vi "Call_enqueue_small.vi"(7 "Waveform":T6(array[cluster])=[{"first point time"=-0.004999939551282051, "xIncrement"=1e-07, "Waveforms"=array[100000 elements]}, {"first point time"=-0.004999939551282051, "xIncrement"=1e-07, "Waveforms"=array[100000 elements]}, {"first point time"=-0.004999939552429668, "xIncrement"=1e-07, "Waveforms"=array[100000 elements]}, {"first point time"=-0.004999939552429668, "xIncrement"=1e-07, "Waveforms"=array[100000 elements]}], 8 "error in":errorcluster, 10 "Input Data":T1 {"Estimate Source" items=["Any Source."=-2, "No Shot"=-1, "Basic Labview Estimate"=0, "IDL Estimate From Andrew"=1, "IDL Estimate From Tobin"=2, "Old Metadata"=3]}, 11 "seconds since 1Jan1904":timestamp=timestamp(3428502400.8921742 s since 1904-01-01)) -> (0 "error IO":errorcluster)   [LabVIEW 2013]
uses:
  Private/Controls/Hardware ID.ctl
  Public API/Dust_Event.ctl
  Public API/Signal.ctl
  Private/Controls/Role ID.ctl
  Private/Controls/Estimate_source.ctl
panel:
  in  "First Detector\nHardware ID":T4=enum."CSA 2"
  in  "Second Detector\nHardware ID":T4=enum."CSA 3"
  # "Dust Event"
  # "Signal"
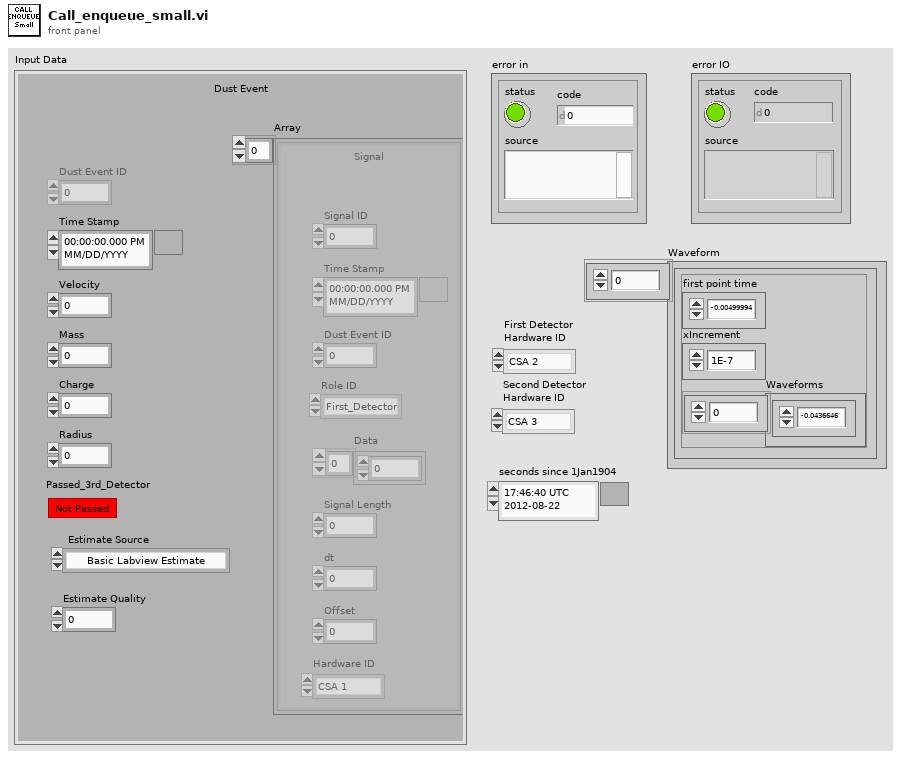
[diagram p1: front panel]
types:
  T1 = typedef "Dust_Event.ctl" = cluster{"Time Stamp":timestamp, "Velocity":sgl, "Mass":sgl, "Charge":sgl, "Radius":sgl, "Array":T2[], "Dust Event ID":i64, "Passed_3rd_Detector":bool, "Estimate Source":T5, "Estimate Quality":sgl}
  T2 = typedef "Signal.ctl" = cluster{"Signal ID":i64, "Time Stamp":timestamp, "Dust Event ID":i64, "Role ID":T3, "Data":sgl[], "Signal Length":i32, "dt":sgl, "Offset":dbl, "Hardware ID":T4}
  T3 = typedef "Role ID.ctl" = enum16{"First_Detector", "Second_Detector", "Third_Detector", "LeCroy_CH1", "LeCroy_CH2", "LeCroy_CH3", "LeCroy_CH4", "PSU"}
  T4 = typedef "Hardware ID.ctl" = enum16{"Unknown", "CSA 1", "CSA 2", "CSA 3", "CSA 4", "CSA 5", "CSA 6"}
  T5 = typedef "Estimate_source.ctl" = i8
  T6 = cluster{"first point time":dbl, "xIncrement":dbl, "Waveforms":dbl[]}[]
  T7 = enum16{"First_Detector", "Second_Detector", "Third_Detector", "LeCroy_CH1", "LeCroy_CH2", "LeCroy_CH3", "LeCroy_CH4"}
  T8 = cluster{"first point time":dbl, "xIncrement":dbl, "Waveforms":dbl[]}
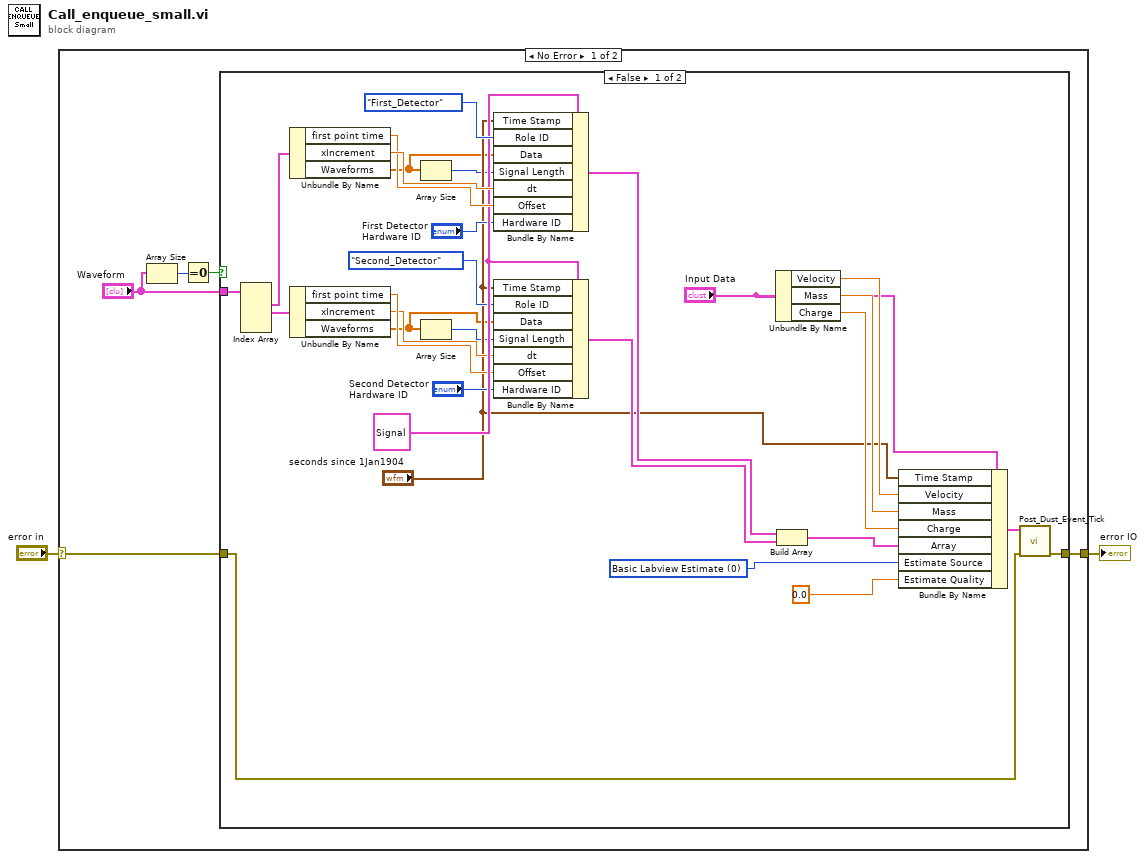
[diagram p0: block diagram]
diagram:
  n1 = case shown="No Error" "error in" {
    selector: "error in" -> [w4 w38]
    tunnel: [w7 w38] -> w1
    frame No Error {
      n2 = Array Size(array="Waveform") -> (size(s)=w6:i32)
      n3 = Equal To 0?(x=w6) -> (x = 0?=w5:bool)
      n4 = case shown="False" w5 {
        tunnel: "Waveform" -> [w35 _]
        tunnel: [w19 w37] -> w7
        tunnel: w4 -> [w18 w37]
        frame False {
          w15 = T5 0 items=["Basic Labview Estimate", "IDL Estimate"] ("Estimate Source")
          w30 = T2 {"Signal ID"=0, "Time Stamp"=timestamp(0 s since 1904-01-01), "Dust Event ID"=0, "Role ID"=enum."First_Detector", "Data"=[], "Signal Length"=0, "dt"=0.0, "Offset"=0.0, "Hardware ID"=enum."CSA 1"} ("Signal")
          n5 = Index Array(array=w35) -> (element #1=w34:T8, element #2=w23:T8)  [unwired: 4 in, 2 out]
          n6 = Unbundle By Name(w34) -> ("first point time"=w32:dbl, "xIncrement"=w33:dbl, "Waveforms"=w11:dbl[])
          n7 = Unbundle By Name(w23) -> ("first point time"=w29:dbl, "xIncrement"=w28:dbl, "Waveforms"=w9:dbl[])
          n8 = Array Size(array=w11) -> (size(s)=w10:i32)
          n9 = Array Size(array=w9) -> (size(s)=w8:i32)
          n10 = Bundle By Name(cluster=w30, "Time Stamp"="seconds since 1Jan1904", "Role ID"=T7."First_Detector", "Data"=w11, "Signal Length"=w10, "dt"=w33, "Offset"=w32, "Hardware ID"="First Detector\nHardware ID") -> (w26:T2)
          n11 = Bundle By Name(cluster=w30, "Time Stamp"="seconds since 1Jan1904", "Role ID"=T7."Second_Detector", "Data"=w9, "Signal Length"=w8, "dt"=w28, "Offset"=w29, "Hardware ID"="Second Detector\nHardware ID") -> (w25:T2)
          n12 = Unbundle By Name("Input Data") -> ("Velocity"=w22:sgl, "Mass"=w21:sgl, "Charge"=w20:sgl)
          n13 = Build Array(w26, w25) -> (w24:T2[])
          n14 = Bundle By Name(cluster="Input Data", "Time Stamp"="seconds since 1Jan1904", "Velocity"=w22, "Mass"=w21, "Charge"=w20, "Array"=w24, "Estimate Source"=w15, "Estimate Quality"=sgl 0.0) -> (w36:T1)
          n15 = call "Post_Dust_Event_Tick.vi"("error in (no error)"=w18, "Input Data"=w36) -> ("error out"=w19:errorcluster)  [unwired: 8 in]
        }
        frame True {
        }
      }
    }
    frame Error {
    }
  }
  "error IO" <- w1
